vi "Read Data Titles.vi"(8 "error in (no error)":errorcluster, 11 "IPS120 in":refnum<class "IPS120.lvclass">) -> (0 "error out":errorcluster, 2 "Data titles":string[](array[string])=["IPS_F (T)"], 3 "IPS120 out":refnum<class "IPS120.lvclass">)   [LabVIEW 2015, in "IPS120.lvclass"]
uses:
  IPS120.lvclass
  ITC503/Controls/ITC503 FP Data.ctl
  OO Devices/Device/Read Controls Snapshot.vi
  OO Devices/Device/Read Control Panel Loaded.vi
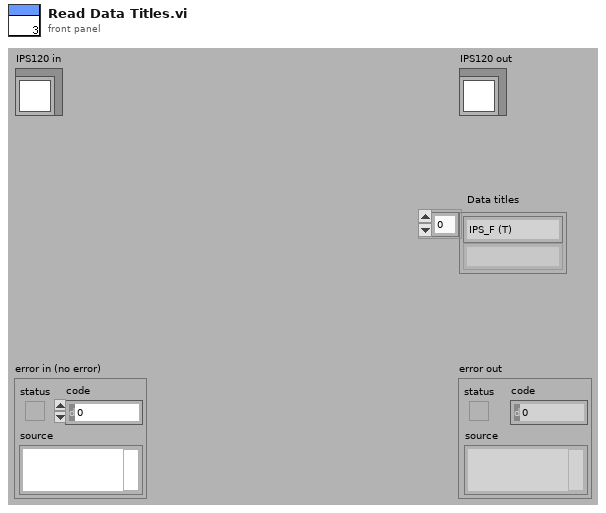
[diagram p1: front panel]
types:
  T1 = typedef "ITC503 FP Data.ctl" = cluster{"Channels to measure":i32[]}
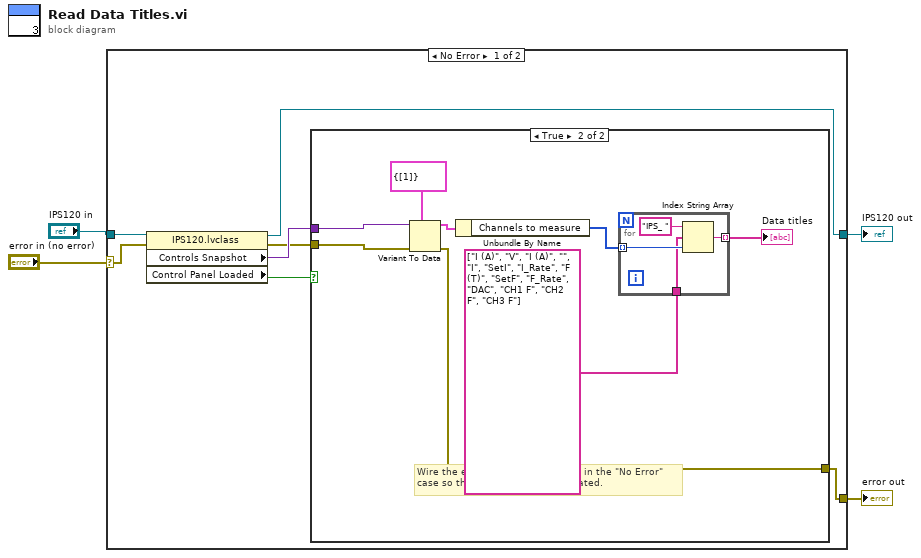
[diagram p0: block diagram]
diagram:
  n1 = case shown="No Error" "error in (no error)" {
    selector: "error in (no error)" -> [w7 w26]
    tunnel: [w5 w26] -> w3
    tunnel: [w6 w25] -> w1
    tunnel: "IPS120 in" -> [w8 w25]
    frame No Error {
      # "Wire the error cluster across even in the \"No Error\"\ncase so that warnings get propagated."
      n2 = property class="IPS120.lvclass"(reference=w8, error in=w7) -> (reference out=w6:refnum<class "IPS120.lvclass">, error out=w10:errorcluster, "Controls Snapshot"=w11:variant, "Control Panel Loaded"=w9:bool)
      n3 = case shown="True" w9 {
        tunnel: w11 -> [_ w20]
        tunnel: w10 -> [w12 w19]
        tunnel: [w12 w13] -> w5
        frame False {
        }
        frame True {
          n4 = Variant To Data(error in=w19, type=T1 {"Channels to measure"=[1]} ("Data"), Variant=w20) -> (data=w17:T1, error out=w13:errorcluster)
          n5 = Unbundle By Name(w17) -> ("Channels to measure"=w16:i32[])
          n6 = for {
            tunnel: w16 -> [w23] mode=indexing
            tunnel: string[] ["I (A)", "V", "I (A)", "", "I", "SetI", "I_Rate", "F (T)", "SetF", "F_Rate", "DAC", "CH1 F", "CH2 F", "CH3 F"] -> [w22]
            tunnel: [w21] -> w14 mode=indexing
            n7 = Index String Array(1:w23, 2:w22, 3:"IPS_ " ("string (\"\")")) -> (0:w21:string)
          }
          "Data titles" <- w14
        }
      }
    }
    frame Error {
    }
  }
  "error out" <- w3
  "IPS120 out" <- w1
